vi "fgt set sensor Unit.vi"(8 "error in (no error)":errorcluster, 10 "unit":T1, 11 "sensorIndex":u32) -> (0 "error out":errorcluster)   [LabVIEW 2020, in "fgt_SDK.lvlib"]
doc: "Set sensor unit on selected sensor device, default value is \"µl/min\" for flowrate sensors and \"mbar\" for pressure sensors.\nEvery sensor read value and regulation command will then use this unit.\nExample of type: \"µl/h\", \"ulperDay\", \"microliter/hour\" ..."
uses:
  fgt_SDK.lvlib
  TypeDefs/fgt_SENSOR_UNIT.ctl
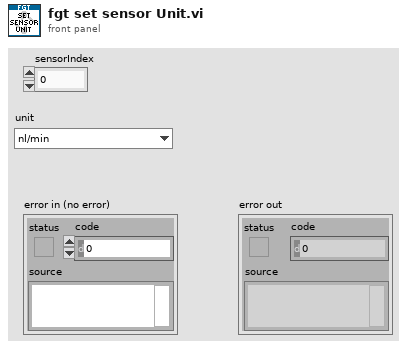
[diagram p1: front panel]
types:
  T1 = typedef "fgt_SDK.lvlib/fgt_SENSOR_UNIT.ctl" = enum16{"nl/min", "µl/s", "µl/min", "ul/h", "ml/min", "ml/h", "mbar", "kPa", "bar"}
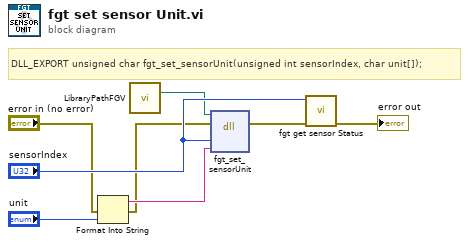
[diagram p0: block diagram]
diagram:
  # "DLL_EXPORT unsigned char fgt_set_sensorUnit(unsigned int sensorIndex, char unit[]);"
  n1 = Format Into String(error in="error in (no error)", "unit") -> (resulting string=w4:string, error out=w2:errorcluster)  [unwired: 2 in]
  n2 = call "LibraryPathFGV.vi"() -> ("Path Out"=w1:path)  [unwired: 14 in, 1 out]
  n3 = dll-call lib="C:/Workspace/fgt-SDK/LabVIEW/dlls/fgt_SDK_*.*" fn="fgt_set_sensorUnit"(path in=w1, error in=w2, "sensorIndex"="sensorIndex", "unit"=w4) -> (error out=w8:errorcluster)  [unwired: 4 in, 1 out]
  n4 = call "fgt get sensor Status.vi"("error in (no error)"=w8, "pressureIndex"="sensorIndex") -> ("error out"=→"error out":errorcluster)  [unwired: 9 in]
